vi "BK Precision 8600 Series Create and Save List File.vi"() -> ()   [LabVIEW 2018]
doc: "Exemplifies how to create a sequence using list mode and saving it into internal memory."
uses:
  <instrlib>/BK Precision 8600 Series/BK Precision 8600 Series.lvlib
panel:
  in  "Range (15)":dbl=15.0001 min=0.0001 max=240.0 step=1.0 format="%.2g"
  in  "VISA resource name":refnum<visa-resource-name>
  in  "Step Level (1)":dbl[](array[numeric]) min=1.0 max=999.99 step=0.01 format="%.4g"
  in  "Step Width (1)":dbl[](array[numeric]) min=2e-05 max=3600.0 step=1.0 format="%.3g"
  in  "Step Slew Rate (0.1)":dbl[](array[numeric]) min=0.0001 max=65536.0 step=0.0001 format="%.4g"
  in  "List Number (1)":dbl=1.0 min=1.0 max=7.0 format="%#_0f"
  in  "Total Steps (2)":dbl=2.0 min=2.0 max=84.0 step=1.0 format="%.0g"
  in  "List Count (1)":dbl=1.0 min=1.0 max=65536.0 step=1.0 format="%.0g"
  in  "Serial Configuration":cluster{"Baud Rate":u32}={"Baud Rate"=9600} {"Baud Rate" items=["300"=300, "600"=600, "1200"=1200, "2400"=2400, "4800"=4800, "9600"=9600, "19200"=19200]}
  # "(c) 2014-2019 B&K Precision Corporation.  ALL RIGHTS RESERVED."
  # "Note:  \n\nList will be saved to List Number location."
  # "Input the step level, width, and slew rate into each index of their respective arrays.  Index 0 is for the first step.  Enter as many step parameter values as needed as specified by Total Steps."
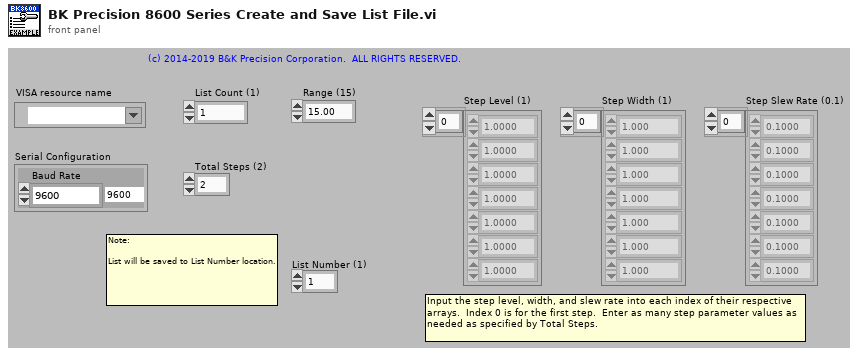
[diagram p1: front panel]
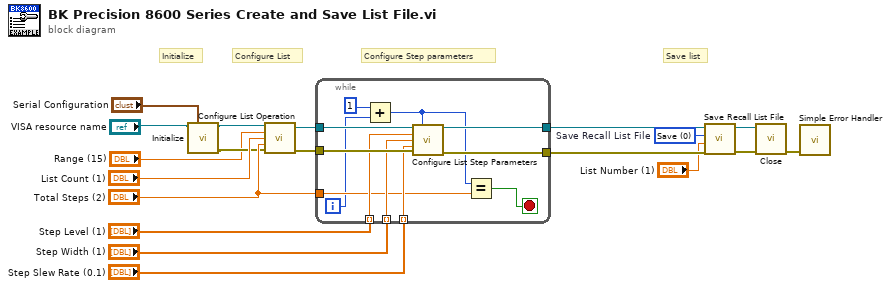
[diagram p0: block diagram]
diagram:
  w6 = u16 0 items=["Save", "Recall"]  # Save Recall List File
  # "Save list"
  # "Configure Step parameters"
  # "Configure List"
  # "Initialize"
  n1 = call <instrlib>:"Initialize.vi"("Serial Configuration"="Serial Configuration", "VISA resource name"="VISA resource name") -> ("error out"=w2:errorcluster, "VISA resource name out"=w3:refnum<visa-resource-name>)  [unwired: 8 in]
  n2 = call <instrlib>:"Configure List Operation.vi"("VISA resource name"=w3, "Range (15)"="Range (15)", "List Count (1)"="List Count (1)", "Total Steps (2)"="Total Steps (2)", "error in (no error)"=w2) -> ("VISA resource name out"=w17:refnum<visa-resource-name>, "error out"=w18:errorcluster)  [unwired: 9 in]
  n3 = while {
    tunnel: w18 -> [w31]
    tunnel: w17 -> [w30]
    tunnel: [w29] -> w16
    tunnel: [w28] -> w15
    tunnel: "Step Level (1)" -> [w27] mode=indexing
    tunnel: "Step Width (1)" -> [w26] mode=indexing
    tunnel: "Step Slew Rate (0.1)" -> [w25] mode=indexing
    tunnel: "Total Steps (2)" -> [w23]
    i -> [w21]
    stop <- w22 stop-if-true
    n4 = Add(x=1, y=w21) -> (x+y=w20:i32)
    n5 = call <instrlib>:"Configure List Step Parameters.vi"("VISA resource name"=w30, "Step Number (1)"=w20, "Step Level (1)"=w27, "Step Width (1)"=w26, "Step Slew Rate (1)"=w25, "error in (no error)"=w31) -> ("VISA resource name out"=w29:refnum<visa-resource-name>, "error out"=w28:errorcluster)  [unwired: 8 in]
    n6 = Equal?(x=w20, y=w23) -> (x = y?=w22:bool)
  }
  n7 = call <instrlib>:"Save Recall List File.vi"("error in (no error)"=w15, "List Number (1)"="List Number (1)", "Save Recall List File (0:Save)"=w6, "VISA resource name"=w16) -> ("error out"=w14:errorcluster, "VISA resource name out"=w13:refnum<visa-resource-name>)  [unwired: 6 in]
  n8 = call <instrlib>:"Close.vi"("error in (no error)"=w14, "VISA resource name"=w13) -> ("error out"=w19:errorcluster)  [unwired: 9 in]
  n9 = call <vilib>:"Simple Error Handler.vi"("error in (no error)"=w19) -> ()  [unwired: 4 in, 5 out]
